vi "init classes.vi"(8 "error in (no error)":errorcluster, 9 "Param Referense":T1, 10 "Data Reference":T2, 11 "Status Reference":T3) -> (0 "error out":errorcluster, 3 "classes":refnum<class "MB_TCP.lvclass">[](array[class]))   [LabVIEW 2019, in "MB_TCP.lvclass"]
uses:
  MB_TCP.lvclass
  Eth Status/Ctl/ICPCON Status.ctl
  MB_TCP_State.ctl
  ICPCON Registers/Ctl/ICPCON Data.ctl
  ICPCON Param/ICPCON Param.ctl
  ICPCON Param/Eth timeouts.ctl
  SMSD/SMSD-DI/SMSD-DI.lvclass
  D:/my_projects/projects/Algorithms/Labview/19/Modbus/MB_TCP2/MB_TCP.lvclass
  SMSD/SMSD-AI/SMSD-AI.lvclass
  ICPCON ET-7024/ICPCON ET-7024.lvclass
  ICPCON ET-7016i/ICPCON ET-7016i.lvclass
  LIR-919D/LIR-919D.lvclass
  TEST/TEST.lvclass
  ICPCON ET-7042i/ICPCON ET-7042i.lvclass
  NS300/NS300.lvclass
  ZERO/ZERO.lvclass
  ICPCON ET-7024i/ICPCON ET-7024i.lvclass
  ICPCON ET-7018i/ICPCON ET-7018i.lvclass
  ICPCON ET-7017/ICPCON ET-7017.lvclass
  ICPCON ET-7051/ICPCON ET-7051.lvclass
  ICPCON ET-7016/ICPCON ET-7016.lvclass
  ICPCON ET-7018/ICPCON ET-7018.lvclass
  MB_TCP.lvclass/MB_TCP.ctl
  Eth Status/Eth Status.lvlib
  ICPCON Registers/ICPCON Registers.lvlib
  ICPCON Param/ICPCON_Param.lvlib
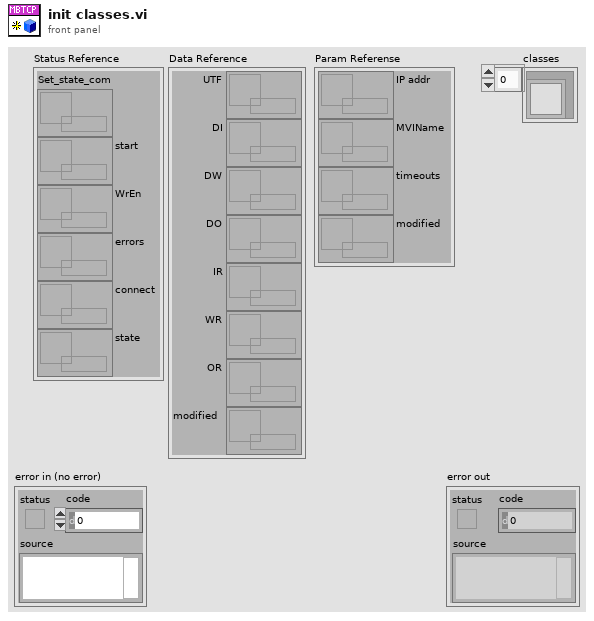
[diagram p1: front panel]
types:
  T1 = typedef "ICPCON_Param.lvlib/ICPCON Param.ctl" = cluster{"IP addr":refnum<data-value>, "MVIName":refnum<data-value>, "timeouts":refnum<data-value>, "modified":refnum<data-value>}
  T2 = typedef "ICPCON Registers.lvlib/ICPCON Data.ctl" = cluster{"UTF":refnum<data-value>, "DI":refnum<data-value>, "DW":refnum<data-value>, "DO":refnum<data-value>, "IR":refnum<data-value>, "WR":refnum<data-value>, "OR":refnum<data-value>, "modified":refnum<data-value>}
  T3 = typedef "Eth Status.lvlib/ICPCON Status.ctl" = cluster{"Set_state_com":refnum<data-value>, "start":refnum<data-value>, "WrEn":refnum<data-value>, "errors":refnum<data-value>, "connect":refnum<data-value>, "state":refnum<data-value>}
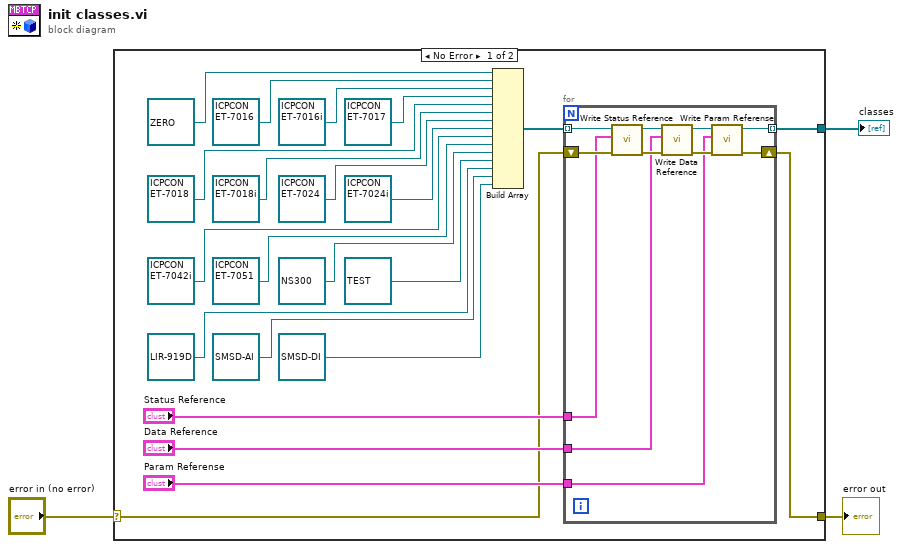
[diagram p0: block diagram]
diagram:
  n1 = case shown="No Error" "error in (no error)" {
    selector: "error in (no error)" -> [w21 w37]
    tunnel: [w20 w37] -> w2
    tunnel: [w22 _] -> w1
    frame No Error {
      n2 = Build Array(refnum<class "ZERO.lvclass"> refnum ("ZERO.lvclass"), refnum<class "ICPCON ET-7016.lvclass"> refnum ("ICPCON ET-7016.lvclass"), refnum<class "ICPCON ET-7016i.lvclass"> refnum ("ICPCON ET-7016i.lvclass"), refnum<class "ICPCON ET-7017.lvclass"> refnum ("ICPCON ET-7017.lvclass"), refnum<class "ICPCON ET-7018.lvclass"> refnum ("ICPCON ET-7018 in"), refnum<class "ICPCON ET-7018i.lvclass"> refnum ("ICPCON ET-7018i.lvclass"), refnum<class "ICPCON ET-7024.lvclass"> refnum ("ICPCON ET-7024.lvclass"), refnum<class "ICPCON ET-7024i.lvclass"> refnum ("ICPCON ET-7024i.lvclass"), refnum<class "ICPCON ET-7042i.lvclass"> refnum ("ICPCON ET-7042i.lvclass"), refnum<class "ICPCON ET-7051.lvclass"> refnum ("ICPCON ET-7051.lvclass"), refnum<class "NS300.lvclass"> refnum ("NS300.lvclass"), refnum<class "TEST.lvclass"> refnum ("TEST.lvclass"), refnum<class "LIR-919D.lvclass"> refnum ("LIR-919D.lvclass"), refnum<class "SMSD-AI.lvclass"> refnum ("SMSD-AI.lvclass"), refnum<class "SMSD-DI.lvclass"> refnum ("SMSD-DI.lvclass")) -> (w4:refnum<class "MB_TCP.lvclass">[])
      n3 = for {
        shift-right: [w30] -> w20
        shift-left: w21 -> [w31]
        tunnel: w4 -> [w32] mode=indexing
        tunnel: "Status Reference" -> [w29]
        tunnel: "Data Reference" -> [w28]
        tunnel: "Param Referense" -> [w27]
        tunnel: [w26] -> w22 mode=indexing
        n4 = call "Write Status Reference.vi"("error in (no error)"=w31, "Status"=w29, "MB_TCP in"=w32) -> ("error out"=w34:errorcluster, "MB_TCP out"=w33:refnum<class "MB_TCP.lvclass">)  [unwired: 7 in]
        n5 = call "Write Data Reference.vi"("error in (no error)"=w34, "Data"=w28, "MB_TCP in"=w33) -> ("error out"=w36:errorcluster, "MB_TCP out"=w35:refnum<class "MB_TCP.lvclass">)  [unwired: 7 in]
        n6 = call "Write Param Referense.vi"("error in (no error)"=w36, "Param Referense"=w27, "MB_TCP in"=w35) -> ("error out"=w30:errorcluster, "MB_TCP out"=w26:refnum<class "MB_TCP.lvclass">)  [unwired: 7 in]
      }
    }
    frame Error {
    }
  }
  "error out" <- w2
  "classes" <- w1
